vi "cblas dger.vi"(0 "x":dbl[](array[numeric]), 1 "y":dbl[](array[numeric]), 2 "A":T2, 3 "alpha":dbl=1.0, 5 "order":T1=101 items=["CblasRowMajor"=101, "CblasColMajor"=102], 8 "lda":i32, 9 "m":i32=-1, 10 "incx":i32=1, 11 "n":i32=-1, 12 "incy":i32=1) -> (14 "dger":T2, 19 "error":i32)   [LabVIEW 2017, in "NI_AALBLAS.lvlib"]
uses:
  NI_AALBLAS.lvlib
  RealMatrix.ctl
  Order.ctl
  NI_Matrix.lvlib
  lvblas.dll
panel:
  # "void cblas_dger(order, m, n, alpha, *x, incx, *y, incy, *A, lda)"
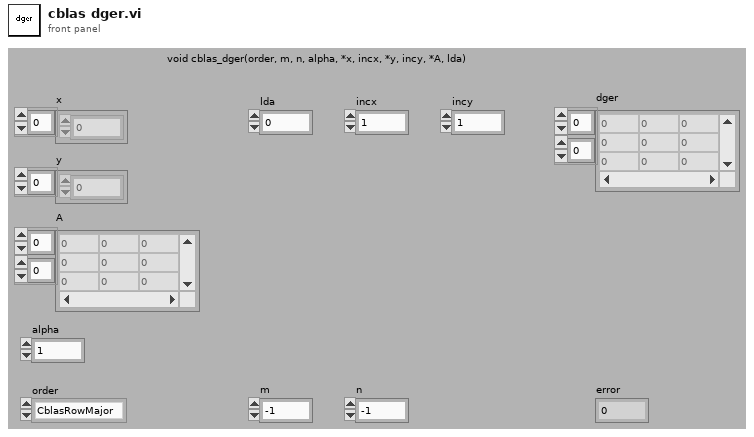
[diagram p1: front panel]
types:
  T1 = typedef "NI_AALBLAS.lvlib/Order.ctl" = i32
  T2 = typedef "NI_Matrix.lvlib/RealMatrix.ctl" = dbl[][]
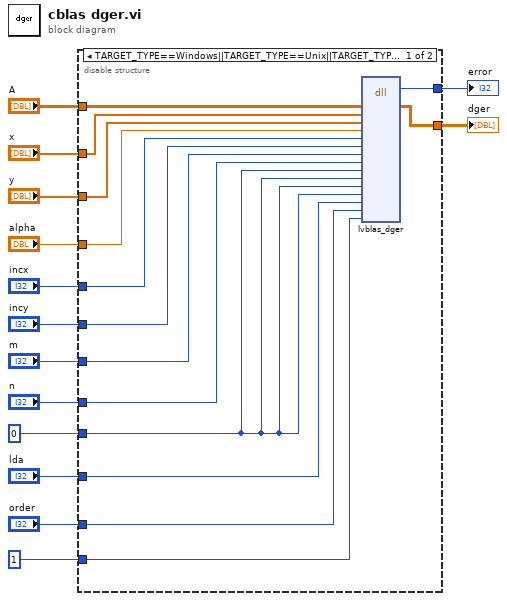
[diagram p0: block diagram]
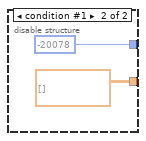
[diagram p2: hidden frame]
diagram:
  n1 = disable-structure shown="TARGET_TYPE==Windows||TARGET_TYPE==Unix||TARGET_TYPE==Mac||TARGET_TYPE==RT" {
    disable-tunnel: "x" -> [w28 _]
    disable-tunnel: "y" -> [w27 _]
    disable-tunnel: "alpha" -> [w26 _]
    disable-tunnel: "A" -> [w25 _]
    disable-tunnel: [w24 -20078 ("error")] -> w10
    disable-tunnel: 0 -> [w23 _]
    disable-tunnel: "lda" -> [w22 _]
    disable-tunnel: [w21 T2 [] ("dger")] -> w7
    disable-tunnel: "order" -> [w20 _]
    disable-tunnel: "incx" -> [w19 _]
    disable-tunnel: "incy" -> [w18 _]
    disable-tunnel: "m" -> [w17 _]
    disable-tunnel: "n" -> [w16 _]
    disable-tunnel: 1 -> [w15 _]
    frame condition #0 (active) {
      n2 = dll-call lib="C:/Program Files/National Instruments/LabVIEW 2017/resource/lvblas.*" fn="lvblas_dger" ("CBLAS.dll:MtrxxVectH")("a"=w25, "x"=w28, "y"=w27, "alpha"=w26, "IncX"=w19, "IncY"=w18, "m"=w17, "n"=w16, "startARow"=w23, "startACol"=w23, "startX"=w23, "startY"=w23, "lda"=w22, "order"=w20, "check"=w15) -> ("error"=w24:i32, "a"=w21:dbl[][])  [unwired: 17 in, 2 out]
    }
    frame condition #1 {
    }
  }
  "dger" <- w7
  "error" <- w10
